vi "First Step.vi"(8 "error in (no error)":errorcluster, 11 "Double Scanner.lvclass in":refnum<class "Double Scanner.lvclass">) -> (0 "error out":errorcluster, 2 "Current Position":dbl, 3 "Double Scanner.lvclass out":refnum<class "Double Scanner.lvclass">)   [LabVIEW 2023, in "Double Scanner.lvclass"]
doc: "(Dynamic) Reset the instrument and prepare to scan. Go to step #0 - the first step. If desired, the scanner may do this in a different way than usual (i.e. by preparing to move a long distance, or reset to home position.)"
uses:
  Double Scanner.lvclass
  Double Scanner.lvclass/Double Scanner.ctl
  Scanner/Scanner.lvclass
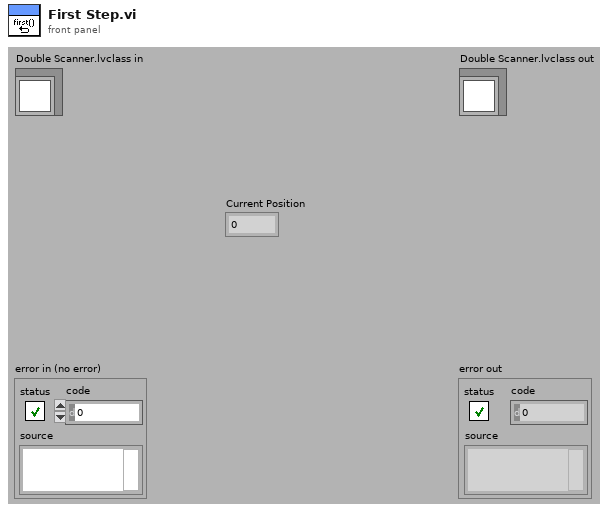
[diagram p1: front panel]
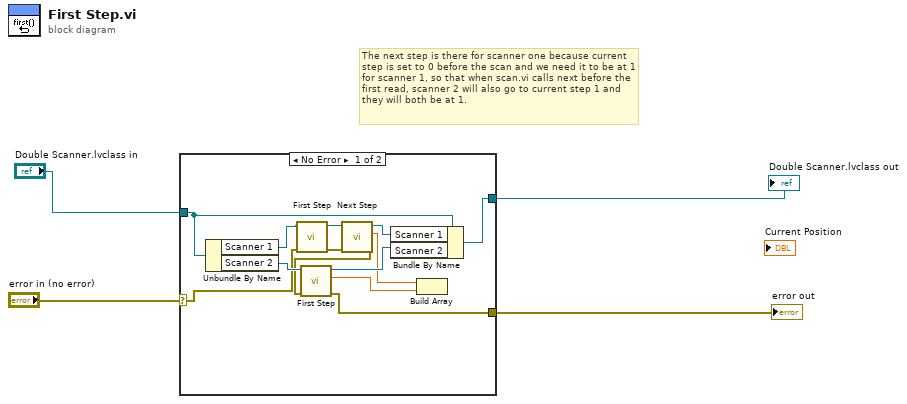
[diagram p0: block diagram]
diagram:
  # "The next step is there for scanner one because current step is set to 0 before the scan and we need it to be at 1 for scanner 1, so that when scan.vi calls next before the first read, scanner 2 will also go to current step 1 and they will both be at 1."
  n1 = case shown="No Error" "error in (no error)" {
    selector: "error in (no error)" -> [w13 w19]
    tunnel: [w12 w19] -> w3
    tunnel: "Double Scanner.lvclass in" -> [w10 w18]
    tunnel: [w11 w18] -> w1
    frame No Error {
      n2 = Unbundle By Name(w10) -> ("Scanner 1"=w14:refnum<class "Scanner.lvclass">, "Scanner 2"=w17:refnum<class "Scanner.lvclass">)
      n3 = call-dynamic "First Step.vi"("error in (no error)"=w13, "Scanner.lvclass in"=w14) -> ("error out"=w7:errorcluster, "Scanner.lvclass out"=w9:refnum<class "Scanner.lvclass">)  [unwired: 7 in, 1 out]
      n4 = call-dynamic "Next Step.vi"("error in (no error)"=w7, "Scanner in"=w9) -> ("error out"=w6:errorcluster, "Current Position"=w5:dbl, "Scanner out"=w8:refnum<class "Scanner.lvclass">)  [unwired: 6 in, 1 out]
      n5 = call-dynamic "First Step.vi"("error in (no error)"=w6, "Scanner.lvclass in"=w17) -> ("error out"=w12:errorcluster, "Current Position"=w15:dbl, "Scanner.lvclass out"=w16:refnum<class "Scanner.lvclass">)  [unwired: 7 in]
      n6 = Bundle By Name(cluster=w10, "Scanner 1"=w8, "Scanner 2"=w16) -> (w11:refnum<class "Double Scanner.lvclass">)
      n7 = Build Array(w5, w15) -> ()  [unwired: 1 out]
    }
    frame Error {
    }
  }
  "error out" <- w3
  "Double Scanner.lvclass out" <- w1
